vi "CreateModesDictionary.vi"(8 "error in (no error)":errorcluster, 11 "Data Value Reference in":T1) -> (0 "error out":errorcluster, 3 "Data Value Reference out":T1)   [LabVIEW 2022 SP3, in "TopLevel.lvclass"]
uses:
  TopLevel.lvclass
  <vilib>/TELLC/Dynamic CVT API/TD Dynamic CVT DVR--ref.ctl
  Common/Controls/DLP_MaterialToHeadMapping--Cluster.ctl
  DLP2/DataTypes/DLP2_PrinterMaterialProperties.ctl
  DLP2/DataTypes/DLP2_PrinterHeadProperties.ctl
  Common/Controls/DLPConfig)Init_HeadPropertyAttr--Cluster.ctl
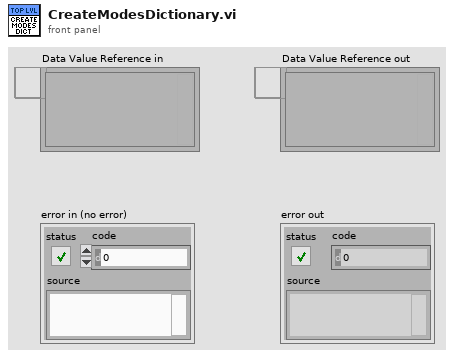
[diagram p1: front panel]
types:
  T1 = typedef "TD Dynamic CVT DVR--ref.ctl" = refnum<data-value>
  T2 = typedef "DLP2_PrinterHeadProperties.ctl" = cluster{"#attributes":T3}
  T3 = typedef "DLPConfig)Init_HeadPropertyAttr--Cluster.ctl" = cluster{"HeadNumber":u8, "Material":string, "HeadLocalX":dbl, "HeadLocalY":dbl, "HeadRotationAngle":dbl, "VH2L_Hi":dbl, "VH2R_Hi":dbl, "VH1LA_Hi":dbl, "VH1LB_Hi":dbl, "VH1RA_Hi":dbl, "VH1RB_Hi":dbl, "VH2L_Lo":dbl, "VH2R_Lo":dbl, "VH1LA_Lo":dbl, "VH1LB_Lo":dbl, "VH1RA_Lo":dbl, "VH1RB_Lo":dbl}
  T4 = typedef "DLP_MaterialToHeadMapping--Cluster.ctl" = cluster{"Head":u8, "Ink":T5}
  T5 = typedef "DLP2_PrinterMaterialProperties.ctl" = cluster{"#attributes":cluster{"InkType":string, "PrePrintPurge":bool, "PurgeTime":dbl, "PurgeCount":i32, "Density":dbl, "NumberofDrops":i32, "PrintWeight":dbl, "PrintheadPrime":bool}, "Idle":cluster{"Name":string, "Heat":dbl, "Meniscus":dbl, "Recirculation":bool}[], "Process":cluster{"Name":string, "Heat":dbl, "Meniscus":dbl, "Recirculation":bool, "ColorPlane":string}[]}
  T6 = cluster{"Name":string, "Heat":dbl, "Meniscus":dbl, "Recirculation":bool}[]
  T7 = cluster{"Name":string, "Heat":dbl, "Meniscus":dbl, "Recirculation":bool, "ColorPlane":string}[]
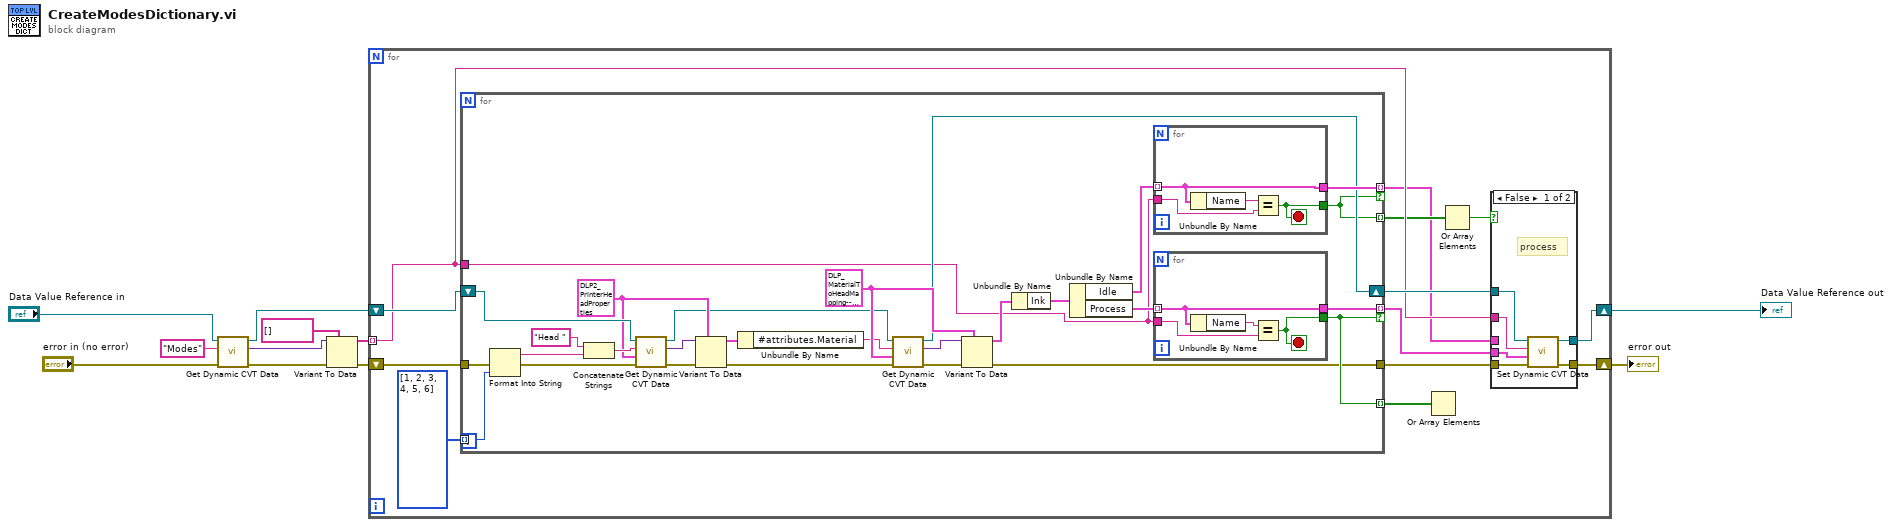
[diagram p0: block diagram]
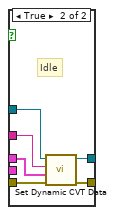
[diagram p2: hidden frame]
diagram:
  n1 = call <vilib>:"Get Dynamic CVT Data.vi"("error in (no error)"="error in (no error)", "DataName"="Modes", "dCVT DVR"="Data Value Reference in") -> ("error out"=w4:errorcluster, "value"=w3:variant, "dCVT DVR out"=w11:T1)  [unwired: 5 in, 1 out]
  n2 = Variant To Data(error in=w4, type=string[] [] ("appended array"), Variant=w3) -> (data=w5:string[], error out=w8:errorcluster)
  n3 = for {
    tunnel: w5 -> [w20] mode=indexing
    shift-right: [w21] -> w6
    shift-left: w11 -> [w23]
    shift-right: [w13] -> w10
    shift-left: w8 -> [w12]
    n4 = for {
      tunnel: i32[] [1, 2, 3, 4, 5, 6] -> [w55] mode=indexing
      tunnel: w20 -> [w41]
      tunnel: [w44] -> w16 mode=indexing if=w40
      tunnel: [w43] -> w15 mode=indexing if=w39
      shift-right: [w42] -> w22
      shift-left: w23 -> [w54]
      tunnel: [w40] -> w19 mode=indexing
      tunnel: [w39] -> w18 mode=indexing
      tunnel: [w38] -> w14
      tunnel: w12 -> [w37]
      w51 = T2 {"#attributes"={"HeadNumber"=0, "Material"="", "HeadLocalX"=0.0, "HeadLocalY"=0.0, "HeadRotationAngle"=0.0, "VH2L_Hi"=0.0, "VH2R_Hi"=0.0, "VH1LA_Hi"=0.0, "VH1LB_Hi"=0.0, "VH1RA_Hi"=0.0, "VH1RB_Hi"=0.0, "VH2L_Lo"=0.0, "VH2R_Lo"=0.0, "VH1LA_Lo"=0.0, "VH1LB_Lo"=0.0, "VH1RA_Lo"=0.0, "VH1RB_Lo"=0.0}} ("HeadProperties")
      w64 = T4 {"Head"=0, "Ink"={"#attributes"={"InkType"="", "PrePrintPurge"=FALSE, "PurgeTime"=0.0, "PurgeCount"=0, "Density"=0.0, "NumberofDrops"=0, "PrintWeight"=0.0, "PrintheadPrime"=FALSE}, "Idle"=[], "Process"=[]}}
      n5 = Format Into String(error in=w37, w55) -> (resulting string=w57:string, error out=w47:errorcluster)  [unwired: 2 in]
      n6 = Concatenate Strings("Head " ("string"), w57) -> (w53:string)
      n7 = call <vilib>:"Get Dynamic CVT Data.vi"("error in (no error)"=w47, "default value (empty variant)"=w51, "DataName"=w53, "dCVT DVR"=w54) -> ("error out"=w50:errorcluster, "value"=w52:variant, "dCVT DVR out"=w45:T1)  [unwired: 4 in, 1 out]
      n8 = Variant To Data(error in=w50, type=w51, Variant=w52) -> (data=w49:T2, error out=w46:errorcluster)
      n9 = Unbundle By Name(w49) -> ("#attributes.Material"=w48:string)
      n10 = call <vilib>:"Get Dynamic CVT Data.vi"("error in (no error)"=w46, "default value (empty variant)"=w64, "DataName"=w48, "dCVT DVR"=w45) -> ("error out"=w62:errorcluster, "value"=w63:variant, "dCVT DVR out"=w42:T1)  [unwired: 4 in, 1 out]
      n11 = Variant To Data(error in=w62, type=w64, Variant=w63) -> (data=w61:T4, error out=w38:errorcluster)
      n12 = Unbundle By Name(w61) -> ("Ink"=w60:T5)
      n13 = Unbundle By Name(w60) -> ("Idle"=w59:T6, "Process"=w58:T7)
      n14 = for {
        tunnel: w59 -> [w71] mode=indexing
        tunnel: w41 -> [w72]
        tunnel: [w69] -> w40
        tunnel: [w71] -> w44
        stop <- w69 stop-if-true
        n15 = Unbundle By Name(w71) -> ("Name"=w70:string)
        n16 = Equal?(x=w70, y=w72) -> (x = y?=w69:bool)
      }
      n17 = for {
        tunnel: w58 -> [w67] mode=indexing
        tunnel: w41 -> [w68]
        tunnel: [w67] -> w43
        tunnel: [w65] -> w39
        stop <- w65 stop-if-true
        n18 = Unbundle By Name(w67) -> ("Name"=w66:string)
        n19 = Equal?(x=w66, y=w68) -> (x = y?=w65:bool)
      }
    }
    n20 = Or Array Elements(Boolean array=w18) -> ()  [unwired: 1 out]
    n21 = Or Array Elements(Boolean array=w19) -> (logical OR=w17:bool)
    n22 = case shown="False" w17 {
      tunnel: w22 -> [w30 w36]
      tunnel: [w29 w35] -> w21
      tunnel: w20 -> [w28 w34]
      tunnel: w16 -> [_ w33]
      tunnel: w15 -> [w27 _]
      tunnel: w14 -> [w26 w32]
      tunnel: [w25 w31] -> w13
      frame False {
        # "process"
        n23 = call <vilib>:"Set Dynamic CVT Data.vi"("error in (no error)"=w26, "value"=w27, "DataName"=w28, "dCVT DVR"=w30) -> ("error out"=w25:errorcluster, "dCVT DVR out"=w29:T1)  [unwired: 5 in, 1 out]
      }
      frame True {
        # "Idle"
        n24 = call <vilib>:"Set Dynamic CVT Data.vi"("error in (no error)"=w32, "value"=w33, "DataName"=w34, "dCVT DVR"=w36) -> ("error out"=w31:errorcluster, "dCVT DVR out"=w35:T1)  [unwired: 5 in, 1 out]
      }
    }
  }
  "error out" <- w10
  "Data Value Reference out" <- w6
